vi "HFRR ADV v021 new software.vi"() -> ()   [LabVIEW 2025] (continued)
          tunnel: w1649 -> [w1703 w1716]
          tunnel: w1648 -> [w1702 w1715]
          tunnel: w1647 -> [_ w1714]
          tunnel: w1645 -> [w1688 w1713]
          tunnel: w1644 -> [w1687 w1712]
          tunnel: w1643 -> [w1686 w1711]
          tunnel: [w1688 w1710] -> w1642
          tunnel: [w1687 w1709] -> w1641
          tunnel: [w1686 w1708] -> w1640
          frame False {
          }
          frame True {
            n1436 = Tick Count (ms)() -> (millisecond timer value=w1745:u32)
            n1437 = String To Byte Array(string=w1714) -> (unsigned byte array=w1758:u8[])
            n1438 = Array Size(array=w1758) -> (size(s)=w1757:i32)
            n1439 = formula code="// --- INTERNAL VARIABLE DECLARATIONS ---\nint i = 0;\nint k = 0;\nint start_idx = -1;\nint end_idx = -1;\nint phase = 0;\nint sign0 = 1;\nint sign1 = 1;\nint ch0_val = 0;   \nint ch1_val = 0;   \nfloat ch0_raw = 0.0;\nfloat ch1_raw = 0.0;\nfloat temp0 = 0.0;\nfloat temp1 = 0.0;\nfloat ch0_clean = 0.0;\nfloat ch1_clean = 0.0;\n\n// Temporal intermediate variables for calculation smoothing\nfloat raw_p2p_v = 0.0;\nfloat raw_friction = 0.0;\nfloat raw_cof = 0.0;\n\n// Initialize output variables to current shift register states right away\nout_LVDT_Min_V = in_LVDT_Min_V;\nout_LVDT_Max_V = in_LVDT_Max_V;\nout_LVDT_P2P_V = in_LVDT_P2P_V;\nout_Piezo_P2P = in_Piezo_P2P;\nout_Friction_N = in_Friction_N;\nout_COF = in_COF;\nwindow_ready = 0;\n\n// --- STEP 1: PARSE EVERY STRING IN THE BYTE ARRAY ---\nif (array_size > 2) {\n    for (i = 0; i < array_size - 1; i++) {\n        if (raw_bytes[i] == 42) { // '*' character detected\n            start_idx = i;\n        }\n        \n        // Match standard delimiter sequence \";&\" or end window character\n        if (raw_bytes[i] == 59 && raw_bytes[i+1] == 38 && start_idx != -1) { \n            end_idx = i;\n            ch0_val = 0;\n            ch1_val = 0;\n            sign0 = 1;\n            sign1 = 1;\n            phase = 0; \n\n            for (k = start_idx + 1; k < end_idx; k++) {\n                if (raw_bytes[k] == 45) { // '-' sign\n                    if (phase == 0) sign0 = -1;\n                    else sign1 = -1;\n                }\n                else if (raw_bytes[k] == 43) { // '+' sign\n                    if (phase == 0) sign0 = 1;\n                    else sign1 = 1;\n                }\n                else if (raw_bytes[k] == 59) { // ';' delimiter\n                    phase = 1; \n                }\n                else if (raw_bytes[k] >= 48 && raw_bytes[k] <= 57) { // Numeric ASCII digits\n                    if (phase == 0) {\n                        ch0_val = (ch0_val * 10) + (raw_bytes[k] - 48);\n                    } else {\n                        ch1_val = (ch1_val * 10) + (raw_bytes[k] - 48);\n                    }\n                }\n            }\n\n            // Implicit type conversion\n            ch0_raw = ch0_val * sign0 * 1.0;\n            ch1_raw = ch1_val * sign1 * 1.0;\n\n            // --- STEP 2: 3-SAMPLE MEDIAN FILTER ---\n            m0_2 = m0_1; m0_1 = m0_0; m0_0 = ch0_raw;\n            float s0_0 = m0_0; float s0_1 = m0_1; float s0_2 = m0_2;\n            if (s0_0 > s0_1) { temp0 = s0_0; s0_0 = s0_1; s0_1 = temp0; }\n            if (s0_1 > s0_2) { temp0 = s0_1; s0_1 = s0_2; s0_2 = temp0; }\n            if (s0_0 > s0_1) { temp0 = s0_0; s0_0 = s0_1; s0_1 = temp0; }\n            ch0_clean = s0_1;\n\n            m1_2 = m1_1; m1_1 = m1_0; m1_0 = ch1_raw;\n            float s1_0 = m1_0; float s1_1 = m1_1; float s1_2 = m1_2;\n            if (s1_0 > s1_1) { temp1 = s1_0; s1_0 = s1_1; s1_1 = temp1; }\n            if (s1_1 > s1_2) { temp1 = s1_1; s1_1 = s1_2; s1_2 = temp1; }\n            if (s1_0 > s1_1) { temp1 = s1_0; s1_0 = s1_1; s1_1 = temp1; }\n            ch1_clean = s1_1;\n\n            // --- STEP 3: EXPONENTIAL FILTER (STREAM LEVEL) ---\n            if (ch0_filt == 0.0) ch0_filt = ch0_clean;\n            if (ch1_filt == 0.0) ch1_filt = ch1_clean;\n\n            ch0_filt = ch0_filt + (ch0_clean - ch0_filt) * 0.125;\n            ch1_filt = ch1_filt + (ch1_clean - ch1_filt) * 0.125;\n\n            // --- STEP 4: MIN/MAX WINDOW CONTINUOUS ACCUMULATION ---\n            if (ch0_filt > max_ch0) max_ch0 = ch0_filt;\n            if (ch0_filt < min_ch0) min_ch0 = ch0_filt;\n            if (ch1_filt > max_ch1) max_ch1 = ch1_filt;\n            if (ch1_filt < min_ch1) min_ch1 = ch1_filt;\n\n            start_idx = -1; \n        }\n    }\n}\n\n// --- STEP 5: WINDOW EVALUATION ENGINE ---\nif (((current_time_ms - start_time_ms) >= 50) && (min_ch0 < 9000000.0) && (max_ch0 > -9000000.0)) {\n    window_ready = 1;\n\n    // Linear Bit-to-Voltage Transformations\n    out_LVDT_Min_V = (min_ch0 * VREF) / 8388607.0;\n    out_LVDT_Max_V = (max_ch0 * VREF) / 8388607.0;\n    raw_p2p_v = out_LVDT_Max_V - out_LVDT_Min_V;\n\n    // Piezo scaling calculations\n    out_Piezo_P2P = max_ch1 - min_ch1;\n    raw_friction = out_Piezo_P2P * PIEZO_CAL_FACTOR;\n    raw_cof = raw_friction / NORMAL_FORCE;\n\n    // --- STEP 6: OUTPUT METRIC SMOOTHING (Low-Pass Filter Alpha = 0.20) ---\n    // Seed initial historical metrics if first loop iteration\n    if (hist_LVDT_P2P == 0.0) hist_LVDT_P2P = raw_p2p_v;\n    if (hist_Friction == 0.0) hist_Friction = raw_friction;\n    if (hist_COF == 0.0)      hist_COF = raw_cof;\n\n    // Apply exponential output dampening\n    hist_LVDT_P2P = hist_LVDT_P2P + (raw_p2p_v - hist_LVDT_P2P) * 0.05;\n    hist_Friction = hist_Friction + (raw_friction - hist_Friction) * 0.05;\n    hist_COF      = hist_COF + (raw_cof - hist_COF) * 0.05;\n\n    // Direct smoothed parameters out to UI Indicators\n    out_LVDT_P2P_V = hist_LVDT_P2P;\n    out_Friction_N = hist_Friction;\n    out_COF        = hist_COF;\n\n    // Reset tracking targets to extreme boundaries safely\n    min_ch0 = 9999999.0;\n    max_ch0 = -9999999.0;\n    min_ch1 = 9999999.0;\n    max_ch1 = -9999999.0;\n\n    start_time_ms = current_time_ms;\n}"("raw_bytes"=w1758, "array_size"=w1757, "VREF"="VREF", "PIEZO_CAL_FACTOR"="PIEZO_CAL_FACTOR", "NORMAL_FORCE"="NORMAL_FORCE", "min_ch0"=w1753, "max_ch0"=w1752, "min_ch1"=w1751, "max_ch1"=w1750, "current_time_ms"=w1745, "start_time_ms"=w1744, "ch0_filt"=w1742, "ch1_filt"=w1741, "m0_0"=w1738, "m0_1"=w1737, "m0_2"=w1736, "m1_0"=w1735, "m1_1"=w1734, "m1_2"=w1733, "in_LVDT_Min_V"=w1726, "in_LVDT_Max_V"=w1719, "in_LVDT_P2P_V"=w1718, "in_Piezo_P2P"=w1717, "in_Friction_N"=w1716, "in_COF"=w1715, "hist_LVDT_P2P"=w1713, "hist_Friction"=w1712, "hist_COF"=w1711) -> ("window_ready"=→"Valid_data":dbl, "out_LVDT_Min_V"=w1725:dbl, "out_LVDT_Max_V"=w1724:dbl, "out_LVDT_P2P_V"=w1723:dbl, "out_Piezo_P2P"=w1722:dbl, "out_Friction_N"=w1721:dbl, "out_COF"=w1720:dbl, "min_ch0"=w1749:dbl, "max_ch0"=w1748:dbl, "min_ch1"=w1747:dbl, "max_ch1"=w1746:dbl, "start_time_ms"=w1743:u32, "ch0_filt"=w1740:dbl, "ch1_filt"=w1739:dbl, "m0_0"=w1732:dbl, "m0_1"=w1731:dbl, "m0_2"=w1730:dbl, "m1_0"=w1729:dbl, "m1_1"=w1728:dbl, "m1_2"=w1727:dbl, "hist_LVDT_P2P"=w1710:dbl, "hist_Friction"=w1709:dbl, "hist_COF"=w1708:dbl)
            "LVDT MIN" <- w1725
            "LVDT MAX" <- w1724
            "LVDT Peak" <- w1723
            "pizo raw" <- w1722
            "Friction" <- w1721
            "cof" <- w1720
          }
        }
      }
      frame Error {
      }
    }
    n1440 = local read "Quit"() -> (w1639:bool)
  }
  n1441 = disable-structure shown="Disabled" {
    disable-tunnel: errorcluster {"status"=TRUE, "code"=0, "source"="Init"} ("error IO") -> [w1784 _]
    disable-tunnel: [w1782 _] -> w48
    frame Disabled {
      n1442 = while {
        shift-right: [w1800] -> w1786
        shift-left: _ -> [w1791]
        shift-right: [w1799] -> w1785
        shift-left: w1784 -> [w1793]
        tunnel: [w1788] -> w1782
        tunnel: [w1798] -> _
        i -> [w1798]
        stop <- w1788 stop-if-true
        n1443 = local read "Port 1a"() -> (w1794:bool)
        n1444 = local read "Port 3"() -> (w1795:bool)
        n1445 = local read "Com Port 1"() -> (w1792:refnum<visa-resource-name>)
        n1446 = Or(x=w1795, y=w1794) -> (x .or. y?=w1797:bool)
        n1447 = Unbundle(w1793) -> ("status"=→"Port 3":bool)  [unwired: 2 out]
        n1448 = Not Equal?(x=w1792, y=w1791) -> (x != y?=w1789:bool)
        n1449 = case shown="True" w1797 {
          frame False {
            w1803 = TRUE ("Visible")
            n1450 = property on="Port 1a" class="Bool (strict)"("Visible"=w1803) -> ()  [unwired: 2 in, 2 out]
            n1451 = property on="Port 3" class="Bool (strict)"("Visible"=w1803) -> ()  [unwired: 2 in, 2 out]
          }
          frame True {
            w1804 = TRUE ("Visible")
            n1452 = property on="Port 1a" class="Bool (strict)"("Visible"=w1804) -> ()  [unwired: 2 in, 2 out]
            n1453 = property on="Port 3" class="Bool (strict)"("Visible"=w1804) -> ()  [unwired: 2 in, 2 out]
          }
        }
        n1454 = Wait (ms)(milliseconds to wait=u32 40) -> ()  [unwired: 1 out]
        n1455 = case shown="True" w1789 {
          tunnel: [w1801 errorcluster {"status"=TRUE, "code"=0, "source"="Init"} ("error out")] -> w1790
          tunnel: w1793 -> [w1801 _]
          frame False {
          }
          frame True {
          }
        }
        "error out 11" <- w1790
        n1456 = case shown="No Error" w1790 {
          selector: w1790 -> [w1811 w1829]
          tunnel: [w1814 w1833] -> w1800
          tunnel: [w1813 w1827] -> w1799
          tunnel: w1791 -> [w1812 w1831]
          frame No Error {
            n1457 = property class="Instr"(reference=w1812, error in=w1811) -> (reference out=w1809:refnum<visa-resource-name>, error out=w1810:errorcluster, "Serial Settings:Number of Bytes at Serial Port"=w1806:u32)
            n1458 = Greater?(x=w1806, y=u32 5) -> (0:w1805:bool)
            n1459 = Not(x=w1805) -> (.not. x?=→"Port 1a":bool)
            n1460 = while {
              tunnel: [w1822] -> w1813
              tunnel: [w1821] -> w1814
              tunnel: w1810 -> [w1820]
              tunnel: w1809 -> [w1819]
              stop <- TRUE stop-if-true
              n1461 = property class="Instr" props=["Serial Settings:Number of Bytes at Serial Port"](reference=w1819, error in=w1820) -> (reference out=w1824:refnum<visa-resource-name>, error out=w1823:errorcluster)  [unwired: 1 out]
              n1462 = VISA Read(VISA resource name=w1824, byte count=u32 50, error in (no error)=w1823) -> (VISA resource name out=w1821:refnum<visa-resource-name>, read buffer=→"UNI READ":string, error out=w1822:errorcluster)  [unwired: 1 out]
              n1463 = Wait (ms)(milliseconds to wait=u32 5) -> ()  [unwired: 1 out]
            }
          }
          frame Error {
            w1839 = u16 0 items=["None", "XON/XOFF", "RTS/CTS", "XON/XOFF & RTS/CTS", "DTR/DSR", "XON/XOFF & DTR/DSR"] ("flow control (0:none)  2")
            w1837 = u16 10 items=["1.0"=10, "1.5"=15, "2.0"=20] ("stop bits 2")
            w1835 = u16 0 items=["None", "Odd", "Even", "Mark", "Space"] ("parity 2")
            w1836 = u32 10000  # timeout (10sec)
            n1464 = VISA Close(VISA resource name=w1831, error in (no error)=w1829) -> (error out=w1832:errorcluster)
            n1465 = local write "Port 1a"(FALSE ("Port 1a")) -> ()
            n1466 = local read "Com Port 1"() -> (w1826:refnum<visa-resource-name>)
            n1467 = call <vilib>:"Clear Errors.vi"("error in (no error)"=w1832) -> ("error out"=w1830:errorcluster)  [unwired: 5 in, 1 out]
            n1468 = call-poly "VISA Configure Serial Port"("VISA resource name"=w1826, "timeout (10sec)"=w1836, "baud rate (9600)"=u32 250000 ("baud rate  2"), "data bits (8)"=u16 8 ("data bits  2"), "parity (0:none)"=w1835, "error in (no error)"=w1830, "stop bits (10: 1 bit)"=w1837, "flow control (0:none)"=w1839) -> ("VISA resource name out"=w1840:refnum<visa-resource-name>, "error out"=w1841:errorcluster)  [unwired: 6 in]
            n1469 = flat-sequence {
              tunnel: w1840 -> [w1843]
              tunnel: w1841 -> [w1842]
              tunnel: [w1843] -> w1833
              tunnel: [w1842] -> w1827
              frame #0 {
                n1470 = Wait (ms)(milliseconds to wait=u32 50) -> ()  [unwired: 1 out]
              }
            }
            "Residual Uno" <- ""
            "Port 1 Error" <- w1827
          }
        }
        n1471 = local read "Quit"() -> (w1788:bool)
        "Error Uno" <- w1793
      }
      n1472 = VISA Close(VISA resource name=w1786, error in (no error)=w1785) -> (error out=w1783:errorcluster)
      n1473 = call <vilib>:"Clear Errors.vi"("error in (no error)"=w1783) -> ()  [unwired: 5 in, 2 out]
    }
    frame Enabled {
    }
  }
  n1474 = while {
    stop <- w1854 stop-if-true
    # "V0OLTAGE TO STROKE (peice vise calibration)"
    n1475 = local read "LVDT MIN"() -> (w1845:dbl)
    n1476 = Wait (ms)(milliseconds to wait=u32 10) -> ()  [unwired: 1 out]
    n1477 = local read "LVDT Peak"() -> (w1846:dbl)
    n1478 = formula code="// Dynamic Parameterized Linear Interpolation Node\n// Inputs: vpp_val, voltages (Array), distances (Array)\n// Outputs: stroke\n\nint i = 0;\nint segments = 11; // 12 points make 11 interpolation segments\n\n// 1. Lower Boundary Clamp\nif (vpp_val <= voltages[0]) {\n    stroke = distances[0];\n}\n// 2. Upper Boundary Clamp\nelse if (vpp_val >= voltages[segments]) {\n    stroke = distances[segments];\n}\n// 3. Dynamic Segment Search Loop\nelse {\n    stroke = distances[0]; // Fallback baseline\n    for (i = 0; i < segments; i++) {\n        if (vpp_val >= voltages[i] && vpp_val <= voltages[i+1]) {\n            // Standard linear interpolation formula using array lookups\n            stroke = distances[i] + (vpp_val - voltages[i]) * (distances[i+1] - distances[i]) / (voltages[i+1] - voltages[i]);\n            break; // Segment found, safely exit the loop\n        }\n    }\n}"("vpp_val"=w1846, "voltages"="calibration values", "distances"="STROKE") -> ("stroke"=→"LVDT STROKE":dbl)
    n1479 = local read "Calibration Tare Value"() -> (w1850:dbl)
    n1480 = local read "Calibration Tare"() -> (w1848:bool)
    n1481 = Subtract(x=w1845, y=w1850) -> (x-y=→"LVDT STROKE  Calibration":dbl)
    n1482 = case shown="True" w1848 {
      selector: w1848 -> [_ w1856]
      tunnel: w1845 -> [_ w1857]
      frame False {
      }
      frame True {
        n1483 = Not(x=w1856) -> (.not. x?=w1855:bool)
        n1484 = local write "Calibration Tare"(w1855) -> ()
        "Calibration Tare Value" <- w1857
      }
    }
    n1485 = local read "Quit"() -> (w1854:bool)
  }
  n1486 = while {
    stop <- w1877 stop-if-true
    n1487 = call <vilib>:"High Resolution Polling Wait.vi"("seconds to wait"=0.02) -> ()  [unwired: 10 in, 1 out]
    n1488 = local read "Due read"() -> (w1875:string)
    n1489 = Spreadsheet String To Array(delimiter (Tab)=";", format string="", spreadsheet string=w1875, array type (2D Dbl)=string[] []) -> (array=w1872:string[])
    n1490 = Fract/Exp String To Number(string=w1872) -> (number=w1871:dbl[])  [unwired: 3 in, 1 out]
    n1491 = Index Array(array=w1871) -> (element #1=→"Sample Temperature":dbl, element #2=→"Target Sample Temperature":dbl, element #3=→"Current Duty Cycle":dbl, element #4=→"Ambient Temperature":dbl, element #5=→"Dac Status":dbl, element #6=→"Vpp":dbl, element #7=→"Active Error Code":dbl, element #8=→"Kp":dbl, element #9=→"Ki":dbl, element #10=→"Kd":dbl, element #11=→"SampleRaw":dbl, element #12=→"AmbRaw":dbl)  [unwired: 12 in]
    n1492 = local read "Quit"() -> (w1877:bool)
  }
  n1493 = while {
    shift-right: [w1891] -> w43
    shift-left: _ -> [w1882]
    shift-right: [w1890] -> w42
    shift-left: errorcluster {"status"=FALSE, "code"=0, "source"="Init"} ("error out") -> [w1884]
    tunnel: [w1879] -> w47
    tunnel: [w1889] -> _
    i -> [w1889]
    stop <- w1879 stop-if-true
    n1494 = local read "Com Port 2"() -> (w1883:refnum<visa-resource-name>)
    n1495 = local read "Port 2a"() -> (w1885:bool)
    n1496 = Unbundle(w1884) -> ("status"=→"Port 4":bool)  [unwired: 2 out]
    n1497 = call <vilib>:"High Resolution Polling Wait.vi"("seconds to wait"=0.02) -> ()  [unwired: 10 in, 1 out]
    n1498 = local read "Port 4"() -> (w1886:bool)
    n1499 = Not Equal?(x=w1883, y=w1882) -> (x != y?=w1881:bool)
    n1500 = Or(x=w1886, y=w1885) -> (x .or. y?=w1888:bool)
    n1501 = case shown="False" w1888 {
      frame False {
        w1894 = TRUE ("Visible")
        n1502 = property on="Port 2a" class="Bool (strict)"("Visible"=w1894) -> ()  [unwired: 2 in, 2 out]
        n1503 = property on="Port 4" class="Bool (strict)"("Visible"=w1894) -> ()  [unwired: 2 in, 2 out]
      }
      frame True {
        w1895 = TRUE ("Visible")
        n1504 = property on="Port 2a" class="Bool (strict)"("Visible"=w1895) -> ()  [unwired: 2 in, 2 out]
        n1505 = property on="Port 4" class="Bool (strict)"("Visible"=w1895) -> ()  [unwired: 2 in, 2 out]
      }
    }
    n1506 = case shown="True" w1881 {
      tunnel: [w1892 errorcluster {"status"=TRUE, "code"=0, "source"="Init"} ("error out")] -> w1880
      tunnel: w1884 -> [w1892 _]
      frame False {
      }
      frame True {
      }
    }
    n1507 = case shown="No Error" w1880 {
      selector: w1880 -> [w1908 w1939]
      tunnel: [w1901 w1944] -> w1891
      tunnel: [w1909 w1937] -> w1890
      tunnel: w1882 -> [w1910 w1942]
      frame No Error {
        n1508 = property class="Instr" props=["Serial Settings:Number of Bytes at Serial Port"](reference=w1910, error in=w1908) -> (reference out=w1902:refnum<visa-resource-name>, error out=w1907:errorcluster)  [unwired: 1 out]
        n1509 = while {
          tunnel: [w1918] -> w1903
          tunnel: [w1917] -> w1904
          tunnel: w1907 -> [w1916]
          tunnel: w1902 -> [w1915]
          tunnel: [w1914] -> _
          i -> [w1914]
          stop <- TRUE stop-if-true
          n1510 = property class="Instr" props=["Serial Settings:Number of Bytes at Serial Port"](reference=w1915, error in=w1916) -> (reference out=w1920:refnum<visa-resource-name>, error out=w1919:errorcluster)  [unwired: 1 out]
          n1511 = VISA Read(VISA resource name=w1920, byte count=u32 1000, error in (no error)=w1919) -> (VISA resource name out=w1917:refnum<visa-resource-name>, read buffer=→"Due read":string, error out=w1918:errorcluster)  [unwired: 1 out]
        }
        n1512 = local read "Command"() -> (w1900:string)
        n1513 = call <vilib>:"Trim Whitespace.vi"("string"=w1900) -> ("trimmed string"=w1899:string)  [unwired: 1 in]
        n1514 = Not Equal?(x=w1899, y="") -> (x != y?=w1905:bool)
        n1515 = VISA Flush I/O Buffer(VISA resource name=w1904) -> (VISA resource name out=w1897:refnum<visa-resource-name>, error out=→"error out 10":errorcluster)  [unwired: 2 in]
        n1516 = case shown="True" w1905 {
          tunnel: w1897 -> [w1922 w1927]
          tunnel: [w1922 w1931] -> w1901
          tunnel: w1903 -> [w1921 w1926]
          tunnel: [w1921 w1929] -> w1909
          tunnel: w1899 -> [_ w1925]
          tunnel: [_ w1928] -> _
          frame False {
            # "DATA  WRITE LOOP"
          }
          frame True {
            n1517 = Concatenate Strings(w1925, "\r\n") -> (w1924:string)
            n1518 = VISA Write(VISA resource name=w1927, write buffer=w1924, error in (no error)=w1926) -> (VISA resource name out=w1931:refnum<visa-resource-name>, return count=w1928:u32, error out=w1930:errorcluster)
            n1519 = flat-sequence {
              tunnel: w1930 -> [w1933]
              tunnel: [w1933] -> w1929
              frame #0 {
                n1520 = local write "Command"("" ("Command")) -> ()
                n1521 = Wait (ms)(milliseconds to wait=u32 5) -> ()  [unwired: 1 out]
              }
            }
          }
        }
        "Port 2a" <- TRUE ("Port 2a")
      }
      frame Error {
        w1950 = u16 0 items=["None", "XON/XOFF", "RTS/CTS", "XON/XOFF & RTS/CTS", "DTR/DSR", "XON/XOFF & DTR/DSR"] ("flow control (0:none)  2")
        w1948 = u16 10 items=["1.0"=10, "1.5"=15, "2.0"=20] ("stop bits 2")
        w1946 = u16 0 items=["None", "Odd", "Even", "Mark", "Space"] ("parity 2")
        w1947 = u32 10000  # timeout (10sec)
        n1522 = VISA Clear(VISA resource name=w1942, error in (no error)=w1939) -> (VISA resource name out=w1941:refnum<visa-resource-name>, error out=w1940:errorcluster)
        n1523 = VISA Close(VISA resource name=w1941, error in (no error)=w1940) -> (error out=w1943:errorcluster)
        n1524 = call <vilib>:"Clear Errors.vi"("error in (no error)"=w1943) -> ()  [unwired: 5 in, 2 out]
        n1525 = local write "Port 2a"(FALSE ("Port 2a")) -> ()
        n1526 = local read "Com Port 2"() -> (w1936:refnum<visa-resource-name>)
        "visa due" <- w1936
        n1527 = call-poly "VISA Configure Serial Port"("VISA resource name"=w1936, "timeout (10sec)"=w1947, "baud rate (9600)"=u32 250000 ("baud rate  2"), "data bits (8)"=u16 8 ("data bits  2"), "parity (0:none)"=w1946, "stop bits (10: 1 bit)"=w1948, "flow control (0:none)"=w1950) -> ("VISA resource name out"=w1951:refnum<visa-resource-name>, "error out"=w1952:errorcluster)  [unwired: 7 in]
        n1528 = flat-sequence {
          tunnel: w1951 -> [w1954]
          tunnel: w1952 -> [w1953]
          tunnel: [w1954] -> w1944
          tunnel: [w1953] -> w1937
          frame #0 {
            n1529 = Wait (ms)(milliseconds to wait=u32 50) -> ()  [unwired: 1 out]
          }
        }
        "Residual Due" <- ""
        "Port 2 Error" <- w1937
      }
    }
    n1530 = local read "Quit"() -> (w1879:bool)
    "Error Due" <- w1884
  }
  n1531 = local write "FRICVALZ"(0.0 ("FRICVALZ")) -> ()
  n1532 = property on="RUN" class="Bool (strict)"("Visible"=TRUE) -> ()  [unwired: 2 in, 2 out]
  n1533 = while {
    tunnel: [w1971] -> _
    tunnel: [w1956] -> w57
    i -> [w1971]
    stop <- w1956 stop-if-true
    n1534 = local read "conststatus"() -> (w1960:dbl)
    n1535 = local read "Main Tab"() -> (w1958:T2)
    n1536 = local read "EDIT"() -> (w1977:bool)
    n1537 = local read "Rate"() -> (w1976:dbl)
    n1538 = case shown="True" w1977 {
      tunnel: [FALSE TRUE] -> w1963
      frame False {
      }
      frame True {
      }
    }
    n1539 = property on="Time slide" class="Slide (strict)"("Scale.Range:Maximum"=2500.0) -> ()  [unwired: 2 in, 2 out]
    n1540 = Equal?(x=w1958, y=T27."About" ("Main Tab")) -> (x = y?=w1969:bool)
    n1541 = Equal?(x=w1960, y=0.0) -> (x = y?=w1961:bool)
    n1542 = Divide(x=1.0, y=w1976) -> (x/y=w1972:dbl)
    "Time 2" <- w1972
    n1543 = case shown="True" w1961 {
      frame False {
      }
      frame True {
        # "C:\\WinDucom\\calibrate WO 2391.dcf"
        n1544 = local write "Lan flag"(22) -> ()
        n1545 = local write "conststatus"(10.0 ("rpm value : 2")) -> ()
        n1546 = String To Path(string="C:\\LAB-IQ\\calibrate WO 2465.dcf") -> (path=w1983:path)
        n1547 = Open/Create/Replace File "Open File"(file path (use dialog)=w1983) -> (refnum out=w1981:refnum<file>)  [unwired: 5 in, 2 out]
        n1548 = for {
          N: 23 -> [_]
          tunnel: w1981 -> [w1992]
          i -> [w1986]
          (unwired) TRUE ("line mode (F)")
          n1549 = Read from Text File "Read File"(file (use dialog)=w1992) -> (text=w1991:string)  [unwired: 3 in, 3 out]
          n1550 = Match Pattern(string=w1991, regular expression="]") -> (after substring=w1989:string)  [unwired: 1 in, 3 out]
          n1551 = String Subset(string=w1991, offset (0)=5, length (rest)=10 ("length (rest)")) -> (substring=w1984:string)
          n1552 = Fract/Exp String To Number(string=w1984) -> (number=w1985:dbl)  [unwired: 3 in, 1 out]
          n1553 = Match Pattern(string=w1989, regular expression="-") -> (before substring=w1987:string)  [unwired: 1 in, 3 out]
          n1554 = case shown="4" w1986 {
            tunnel: w1985 -> [w1995 w1996 w1997 w1998 _ _ _ w2003 w2004 _ w2005 w2006 w2007 w2008 w2009 w2010 _ w2011 w2012 _ _ _ _ _]
            tunnel: w1987 -> [_ _ _ _ w1999 w2000 w2001 _ _ _ _ _ _ _ _ _ _ _ _ w2013 w2014 w2015 w2016 _]
            frame 0 {
              n1555 = local write "FRIC. FORCE :"(w1995) -> ()
            }
            frame 1 {
              n1556 = local write "TEMPERATURE :"(w1996) -> ()
            }
            frame 2 {
              n1557 = local write "HUMIDITY:"(w1997) -> ()
            }
            frame 3 {
              n1558 = local write "AIR TEMPERATURE :"(w1998) -> ()
            }
            frame 4 {
              n1559 = local write "Com Port 1"(w1999) -> ()
            }
            frame 5 {
              n1560 = local write "Com Port 2"(w2000) -> ()
              n1561 = local write "visa due"(w2000) -> ()
            }
            frame 6 {
              n1562 = String To Path(string=w2001) -> (path=w2002:path)
              n1563 = local write "File Path"(w2002) -> ()
              "String" <- w2001
            }
            frame 7 {
              n1564 = local write "DISPLACEMENT :"(w2003) -> ()
            }
            frame 8 {
              n1565 = local write "STROKE GAIN :"(w2004) -> ()
            }
            frame 9 {
            }
            frame 10 {
              n1566 = local write "Language Selection"(w2005) -> ()
            }
            frame 11 {
              n1567 = local write "CH-POWER +"(w2006) -> ()
            }
            frame 12 {
              n1568 = local write "CH-POWER -"(w2007) -> ()
            }
            frame 13 {
              n1569 = local write "CH-HEATER"(w2008) -> ()
            }
            frame 14 {
              n1570 = local write "CH-HUMIDITY WET"(w2009) -> ()
            }
            frame 15 {
              n1571 = local write "CH-HUMIDITY DRY"(w2010) -> ()
            }
            frame 16 {
            }
            frame 17 {
              n1572 = local write "AIR TEMP INTERCEPT:"(w2011) -> ()
            }
            frame 18 {
              n1573 = local write "TEMP INTERCEPT:"(w2012) -> ()
            }
            frame 21 {
              n1574 = local write "S.NO"(w2013) -> ()
            }
            frame 22 {
              n1575 = local write "Com Port 3"(w2014) -> ()
            }
            frame 20 {
              n1576 = local write "Camera Port :"(w2015) -> ()
            }
            frame 19 {
              n1577 = local write "C3 :"(w2016) -> ()
            }
            frame 23, Default {
            }
          }
        }
      }
    }
    n1578 = Select(t=u32 2500 ("milliseconds to wait"), s=w1969, f=u32 500 ("milliseconds to wait")) -> (s? t:f=w1967:u32)
    n1579 = Multiply(x=w1972, y=w1967) -> (x*y=w1974:dbl)
    n1580 = property on="Time slide" class="Slide (strict)"("Visible"=w1963) -> ()  [unwired: 2 in, 2 out]
    n1581 = call "Elapsed Time2"("Time Target (s)"=w1974, "Auto Reset"=TRUE) -> ("Time has Elapsed"=w1964:bool)  [unwired: 10 in, 7 out]
    n1582 = case shown="True" w1964 {
      frame False {
      }
      frame True {
        n1583 = stacked-sequence {
          frame #0 {
            # "DATA PROCESSING"
            # "115 mV/N"
            n1584 = local read "Sample Temperature"() -> (w2019:dbl)
            n1585 = local read "RH Numeric:"() -> (w2026:dbl)
            n1586 = local read "HUMIDITY:"() -> (w2027:dbl)
            n1587 = local read "FRICVALZ"() -> (w2038:dbl)
            n1588 = local read "Friction"() -> (w2022:dbl)
            n1589 = Multiply(x=w2026, y=w2027) -> (x*y=→"Humidity ( %RH )" →"Hum" →"Hum 2":dbl)
            n1590 = call <vilib>:"Mean PtByPt.vi"("x"=w2019, "sample length"=100) -> ("mean"=w2018:dbl)  [unwired: 2 in, 1 out]
            "TEMP 2" <- w2018
            "TEMP 3" <- w2018
            n1591 = Subtract(x=w2022, y=w2038) -> (x-y=w2033:dbl)
            "FF 2" <- w2033
            "FF 4" <- w2033
            n1592 = local read "Ambient Temperature"() -> (→"AIR TEMP":dbl)
            n1593 = local read "TEMP"() -> (w2037:dbl)
            n1594 = local write "FF 3"(w2033) -> ()
            n1595 = Compound Arithmetic op=OR("FRICVALZ 4", "FRICVALZ 3", "FRICVALZ 2") -> (w2029:bool)
            n1596 = case shown="True" w2029 {
              tunnel: w2022 -> [_ w2044]
              frame False {
              }
              frame True {
                w2043 = FALSE ("FRICVALZ")
                n1597 = local write "FRICVALZ 3"(w2043) -> ()
                n1598 = local write "FRICVALZ 2"(w2043) -> ()
                n1599 = local write "FRICVALZ 4"(w2043) -> ()
                "FRICVALZ" <- w2044
              }
            }
            n1600 = Not A Number/Path/Refnum?(number/path/refnum=w2037) -> (NaN/Path/Refnum?=w2036:bool)
            n1601 = Not A Number/Path/Refnum?(number/path/refnum=w2033) -> (NaN/Path/Refnum?=w2035:bool)
            n1602 = Divide(x=w2033, y=1.96) -> (x/y=w2030:dbl)
            n1603 = Compound Arithmetic op=OR(w2036, w2035) -> (w2034:bool)
            n1604 = Not A Number/Path/Refnum?(number/path/refnum=w2030) -> (NaN/Path/Refnum?=w2031:bool)
            n1605 = case shown="True" w2034 {
              frame False {
              }
              frame True {
                n1606 = local write "TEMP"(0.0 ("TEMP")) -> ()
                n1607 = local write "FF 2"(0.0 ("FF 2")) -> ()
                n1608 = local write "reinit"(TRUE ("reinit")) -> ()
              }
            }
            n1609 = local write "TEMP"(w2018) -> ()
            n1610 = Select(t=0.0, s=w2031, f=w2030) -> (s? t:f=w2021:dbl)
            "COF 2" <- w2021
            n1611 = local write "COF 3"(w2021) -> ()
          }
        }
      }
    }
    n1612 = Wait (ms)(milliseconds to wait=u32 50) -> ()  [unwired: 1 out]
    n1613 = local read "Quit"() -> (w1956:bool)
    "Rate" <- 2500.0 ("No of Samples")
  }
  n1614 = while {
    tunnel: w60 -> [_]
    tunnel: [w2071] -> _
    tunnel: [w2047] -> w59
    i -> [w2071]
    stop <- w2047 stop-if-true
    # "C:\\LAB-IQ-NXT\\Scar View.exe"
    n1615 = local read "OK Button 16"() -> (w2060:bool)
    n1616 = local read "Main Tab"() -> (w2053:T2)
    n1617 = local read "service 3"() -> (w2054:bool)
    n1618 = local read "OPEN 6"() -> (w2056:bool)
    n1619 = local read "EDIT 2"() -> (w2058:bool)
    n1620 = flat-sequence {
      frame #0 {
        n1621 = local read "SAVE 2"() -> (w2673:bool)
        n1622 = stacked-sequence {
          frame #0 {
            n1623 = local read "EDIT"() -> (w2727:bool)
            n1624 = case shown="True" w2727 {
              tunnel: [u8 2 ("Disabled") u8 0 ("Disabled")] -> _
              frame False {
                w2729 = FALSE
                n1625 = local write "Password"("") -> ()
                n1626 = property on="SrvM CP" class="Bool (strict)"("Visible"=w2729) -> ()  [unwired: 2 in, 2 out]
                n1627 = property on="message" class="Str"("Visible"=w2729) -> ()  [unwired: 2 in, 2 out]
                n1628 = local write "x = y?"(w2729) -> ()
                n1629 = property on="Password" class="Str"("Visible"=w2729) -> ()  [unwired: 2 in, 2 out]
                n1630 = property on="ENTER THE NEW PASSWORD" class="Str"("Visible"=w2729) -> ()  [unwired: 2 in, 2 out]
                n1631 = property on="ENTER CURRENT PASSWORD" class="Str"("Visible"=w2729) -> ()  [unwired: 2 in, 2 out]
                n1632 = local write "SrvM CP"(w2729) -> ()
              }
              frame True {
                w2732 = TRUE
                n1633 = property on="SrvM CP" class="Bool (strict)"("Visible"=w2732) -> ()  [unwired: 2 in, 2 out]
                n1634 = property on="Password" class="Str"("Visible"=w2732) -> ()  [unwired: 2 in, 2 out]
              }
            }
            "dipl pwd" <- "@143$\n" ("dipl pwd")
          }
          frame #1 {
            # "Gain password"
            n1635 = String To Byte Array(string="ENTER CURRENT PASSWORD") -> (unsigned byte array=w2737:u8[])
            n1636 = Search 1D Array(1D array=w2737, element=u8 10) -> (index of element=w2740:i32)  [unwired: 1 in]
            n1637 = Index Array(array=w2737, index=w2740) -> (element=w2736:u8)
            n1638 = Equal?(x=w2736, y=10) -> (x = y?=w2734:bool)
            n1639 = case shown="True" w2734 {
              frame False {
                n1640 = property on="ENTER THE NEW PASSWORD" class="Str"("Visible"=FALSE) -> ()  [unwired: 2 in, 2 out]
              }
              frame True {
                # "password"
                # "change password logic"
                n1641 = local read "ENTER CURRENT PASSWORD"() -> (w2753:string)
                n1642 = local read "dipl pwd"() -> (w2747:string)
                n1643 = String To Byte Array(string=w2753) -> (unsigned byte array=w2755:u8[])
                n1644 = String To Byte Array(string=w2747) -> (unsigned byte array=w2748:u8[])
                n1645 = Array Size(array=w2755) -> (size(s)=w2752:i32)
                n1646 = Array Size(array=w2748) -> (size(s)=w2750:i32)
                n1647 = for {
                  N: w2752 -> [_]
                  tunnel: w2755 -> [w2779]
                  tunnel: [w2777] -> w2756 mode=indexing
                  tunnel: w2752 -> [w2771]
                  i -> [w2772]
                  n1648 = Decrement(x=w2771) -> (x-1=w2769:i32)
                  n1649 = Equal?(x=w2772, y=w2769) -> (x = y?=w2770:bool)
                  n1650 = Index Array(array=w2779, index=w2772) -> (element=w2773:u8)
                  n1651 = Number To Decimal String(number=w2773) -> (decimal integer string=w2778:string)  [unwired: 1 in]
                  n1652 = Select(t="", s=w2770, f="\r") -> (s? t:f=w2775:string)
                  n1653 = Concatenate Strings(w2778, w2775) -> (w2777:string)
                }
                n1654 = for {
                  N: w2750 -> [_]
                  tunnel: w2748 -> [w2767]
                  tunnel: [w2765] -> w2749 mode=indexing
                  tunnel: w2750 -> [w2762]
                  i -> [w2763]
                  n1655 = Decrement(x=w2762) -> (x-1=w2761:i32)
                  n1656 = Equal?(x=w2763, y=w2761) -> (x = y?=w2760:bool)
                  n1657 = Index Array(array=w2767, index=w2763) -> (element=w2766:u8)
                  n1658 = Number To Decimal String(number=w2766) -> (decimal integer string=w2764:string)  [unwired: 1 in]
                  n1659 = Select(t="", s=w2760, f="\r") -> (s? t:f=w2757:string)
                  n1660 = Concatenate Strings(w2764, w2757) -> (w2765:string)
                }
                n1661 = local read "string"() -> (w2754:string)
                n1662 = Concatenate Strings(w2749) -> (w2743:string)
                n1663 = Concatenate Strings(w2754) -> (w2751:string)
                n1664 = Concatenate Strings(w2756) -> (w2744:string)
                n1665 = Equal?(x=w2744, y=w2751) -> (x = y?=w2746:bool)
                n1666 = Equal?(x=w2744, y=w2743) -> (x = y?=w2742:bool)
                n1667 = Or(x=w2746, y=w2742) -> (x .or. y?=w2745:bool)
                n1668 = case shown="True" w2745 {
                  frame False {
                  }
                  frame True {
                    n1669 = property on="ENTER THE NEW PASSWORD" class="Str"("Visible"=TRUE) -> ()  [unwired: 2 in, 2 out]
                  }
                }
              }
            }
          }
          frame #2 {
            n1670 = String To Byte Array(string="ENTER THE NEW PASSWORD") -> (unsigned byte array=w2782:u8[])
            n1671 = Search 1D Array(1D array=w2782, element=u8 10) -> (index of element=w2786:i32)  [unwired: 1 in]
            n1672 = Index Array(array=w2782, index=w2786) -> (element=w2784:u8)
            n1673 = Equal?(x=w2784, y=10) -> (x = y?=w2781:bool)
            n1674 = case shown="False" w2781 {
              frame False {
              }
              frame True {
                n1675 = local write "EDIT"(FALSE) -> ()
                n1676 = local write "SrvM CP"(FALSE) -> ()
                n1677 = local read "ENTER THE NEW PASSWORD"() -> (w2789:string)
                n1678 = String To Byte Array(string=w2789) -> (unsigned byte array=w2794:u8[])
                n1679 = Array Size(array=w2794) -> (size(s)=w2791:i32)
                n1680 = for {
                  N: w2791 -> [_]
                  tunnel: w2794 -> [w2807]
                  tunnel: [w2804] -> w2796 mode=indexing
                  tunnel: w2791 -> [w2799]
                  i -> [w2797]
                  n1681 = Decrement(x=w2799) -> (x-1=w2800:i32)
                  n1682 = Equal?(x=w2797, y=w2800) -> (x = y?=w2801:bool)
                  n1683 = Index Array(array=w2807, index=w2797) -> (element=w2806:u8)
                  n1684 = Number To Decimal String(number=w2806) -> (decimal integer string=w2805:string)  [unwired: 1 in]
                  n1685 = Select(t="", s=w2801, f="\r") -> (s? t:f=w2798:string)
                  n1686 = Concatenate Strings(w2805, w2798) -> (w2804:string)
                }
                n1687 = local read "file path"() -> (w2788:path)
                n1688 = Concatenate Strings(w2796) -> (w2790:string)
                n1689 = Delete(path (use dialog)=w2788) -> (deleted path=w2792:path)  [unwired: 4 in, 2 out]
                n1690 = call <vilib>:"Write Characters To File.vi"("append to file? (new file:F)"=FALSE, "character string"=w2790, "file path (dialog if empty)"=w2792) -> ()  [unwired: 2 in, 1 out]
              }
            }
          }
          frame #3 {
            n1691 = case shown="True" "SrvM CP" {
              frame False {
                w2810 = ""
                n1692 = local write "ENTER CURRENT PASSWORD"(w2810) -> ()
                n1693 = local write "ENTER THE NEW PASSWORD"(w2810) -> ()
                n1694 = property on="ENTER CURRENT PASSWORD" class="Str"("Visible"=FALSE) -> ()  [unwired: 2 in, 2 out]
              }
              frame True {
                n1695 = property on="ENTER THE NEW PASSWORD" class="Str"() -> ("Visible"=w2811:bool)  [unwired: 2 in, 2 out]
                n1696 = Not(x=w2811) -> (.not. x?=w2812:bool)
                n1697 = property on="ENTER CURRENT PASSWORD" class="Str"("Visible"=w2812) -> ()  [unwired: 2 in, 2 out]
              }
            }
          }
          frame #4 {
            n1698 = String To Byte Array(string="Password") -> (unsigned byte array=w2819:u8[])
            n1699 = Search 1D Array(1D array=w2819, element=u8 10) -> (index of element=w2817:i32)  [unwired: 1 in]
            n1700 = Index Array(array=w2819, index=w2817) -> (element=w2818:u8)
            n1701 = Equal?(x=w2818, y=10) -> (x = y?=w2814:bool)
            n1702 = case shown="True" w2814 {
              frame False {
              }
              frame True {
                # "password"
                # "password"
                n1703 = local read "Password"() -> (w2832:string)
                n1704 = String To Byte Array(string=w2832) -> (unsigned byte array=w2835:u8[])
                n1705 = String To Byte Array(string="@143$\n") -> (unsigned byte array=w2821:u8[])
                n1706 = Array Size(array=w2835) -> (size(s)=w2830:i32)
                n1707 = Array Size(array=w2821) -> (size(s)=w2826:i32)
                n1708 = for {
                  N: w2830 -> [_]
                  tunnel: w2835 -> [w2869]
                  tunnel: [w2867] -> w2836 mode=indexing
                  tunnel: w2830 -> [w2864]
                  i -> [w2865]
                  n1709 = Decrement(x=w2864) -> (x-1=w2863:i32)
                  n1710 = Index Array(array=w2869, index=w2865) -> (element=w2868:u8)
                  n1711 = Equal?(x=w2865, y=w2863) -> (x = y?=w2862:bool)
                  n1712 = Number To Decimal String(number=w2868) -> (decimal integer string=w2866:string)  [unwired: 1 in]
                  n1713 = Select(t="", s=w2862, f="\r") -> (s? t:f=w2859:string)
                  n1714 = Concatenate Strings(w2866, w2859) -> (w2867:string)
                }
                n1715 = for {
                  N: w2826 -> [_]
                  tunnel: w2821 -> [w2880]
                  tunnel: [w2878] -> w2824 mode=indexing
                  tunnel: w2826 -> [w2875]
                  i -> [w2876]
                  n1716 = Decrement(x=w2875) -> (x-1=w2874:i32)
                  n1717 = Index Array(array=w2880, index=w2876) -> (element=w2879:u8)
                  n1718 = Equal?(x=w2876, y=w2874) -> (x = y?=w2873:bool)
                  n1719 = Number To Decimal String(number=w2879) -> (decimal integer string=w2877:string)  [unwired: 1 in]
                  n1720 = Select(t="", s=w2873, f="\r") -> (s? t:f=w2870:string)
                  n1721 = Concatenate Strings(w2877, w2870) -> (w2878:string)
                }
                n1722 = local read "file path"() -> (w2820:path)
                n1723 = call <vilib>:"Read Characters From File.vi"("file path (dialog if empty)"=w2820) -> ("character string"=w2834:string)  [unwired: 5 in, 3 out]
                "string" <- w2834
                n1724 = flat-sequence {
                  tunnel: [w2837] -> w2831
                  frame #0 {
                    w2837 = ""
                    n1725 = local write "Password"(w2837) -> ()
                  }
                }
                n1726 = Concatenate Strings(w2824) -> (w2825:string)
                n1727 = Concatenate Strings(w2834) -> (w2833:string)
                n1728 = Concatenate Strings(w2836) -> (w2828:string)
                n1729 = Equal?(x=w2828, y=w2833) -> (x = y?=w2823:bool)
                n1730 = Equal?(x=w2828, y=w2825) -> (x = y?=w2829:bool)
                n1731 = Or(x=w2823, y=w2829) -> (x .or. y?=w2822:bool)
                "x = y?" <- w2822
                n1732 = case shown="True" w2822 {
                  selector: w2822 -> [w2839 _]
                  tunnel: w2831 -> [_ _]
                  frame False {
                    n1733 = And(x=w2839, y=TRUE ("Visible")) -> (x .and. y?=w2840:bool)
                    n1734 = property on="message" class="Str"("Visible"=w2840) -> ()  [unwired: 2 in, 2 out]
                  }
                  frame True {
                    n1735 = control-ref of="This VI"() -> (w2851:refnum<vi>)
                    n1736 = property class="VI"(reference=w2851) -> (reference out=w2842:refnum<vi>, error out=w2846:errorcluster, "Panel"=w2850:refnum<vi>)  [unwired: 1 in]
                    n1737 = property on="message" class="Str"("Visible"=FALSE) -> ()  [unwired: 2 in, 2 out]
                    n1738 = property class="Pnl"(reference=w2850, error in=w2846) -> (reference out=w2844:refnum<vi>, error out=w2847:errorcluster, "Panes[]"=w2849:refnum<vi>[])
                    n1739 = for {
                      tunnel: w2849 -> [w2858] mode=indexing
                      tunnel: T21."Always On" ("Horizontal Scrollbar Visibility") -> [w2857]
                      tunnel: w2847 -> [w2854]
                      tunnel: [w2853] -> w2845
                      n1740 = property class="Pane"(reference=w2858, error in=w2854, "HorizScrollbarVisibility"=w2857) -> (reference out=w2855:refnum<vi>, error out=w2856:errorcluster)
                      n1741 = Close Reference(reference=w2855, error in (no error)=w2856) -> (error out=w2853:errorcluster)
                    }
                    n1742 = Close Reference(reference=w2844, error in (no error)=w2845) -> (error out=w2843:errorcluster)
                    n1743 = Close Reference(reference=w2842, error in (no error)=w2843) -> (error out=→"error out 6":errorcluster)
                  }
                }
              }
            }
          }
        }
        n1744 = local read "x = y?"() -> (w2679:bool)
        n1745 = local read "HUMIDITY: 2"() -> (w2681:dbl)
        n1746 = local read "HUMIDITY:"() -> (w2680:dbl)
        n1747 = property on="Port 2 Error" class="Clust (strict)"("Visible"="EDIT") -> ()  [unwired: 2 in, 2 out]
        n1748 = property on="Port 1 Error" class="Clust (strict)"("Visible"="EDIT") -> ()  [unwired: 2 in, 2 out]
        n1749 = case shown="True" "SrvM CP 2" {
          frame False {
          }
          frame True {
            n1750 = local write "SrvM CP 2"(FALSE ("SrvM CP 2")) -> ()
            n1751 = local read "HUMIDITY: 2"() -> (w2720:dbl)
            n1752 = local read "TEMP INTERCEPT: 2"() -> (w2719:dbl)
            n1753 = local read "DISPLACEMENT : 4"() -> (w2723:dbl)
            n1754 = local read "TEMPERATURE : 2"() -> (w2722:dbl)
            n1755 = local read "STROKE GAIN : 2"() -> (w2724:dbl)
            n1756 = local read "FRIC. FORCE : 2"() -> (w2725:dbl)
            n1757 = local read "AIR TEMP INTERCEPT: 2"() -> (w2718:dbl)
            n1758 = local read "AIR TEMPERATURE : 2"() -> (w2721:dbl)
            n1759 = local write "HUMIDITY:"(w2720) -> ()
            n1760 = local write "AIR TEMP INTERCEPT:"(w2719) -> ()
            n1761 = local write "TEMPERATURE :"(w2722) -> ()
            n1762 = local write "FRIC. FORCE :"(w2725) -> ()
            n1763 = local write "STROKE GAIN :"(w2724) -> ()
            n1764 = local write "DISPLACEMENT :"(w2723) -> ()
            n1765 = local write "AIR TEMPERATURE :"(w2721) -> ()
            n1766 = local write "TEMP INTERCEPT:"(w2718) -> ()
          }
        }
        n1767 = Or(x="SAVE", y=w2673) -> (x .or. y?=w2674:bool)
        n1768 = And(x="EDIT", y=w2679) -> (x .and. y?=w2677:bool)
        n1769 = local read "DISPLACEMENT : 4"() -> (w2690:dbl)
        n1770 = local read "TEMPERATURE : 2"() -> (w2688:dbl)
        n1771 = local read "STROKE GAIN : 2"() -> (w2694:dbl)
        n1772 = local read "DISPLACEMENT :"() -> (w2689:dbl)
        n1773 = local read "FRIC. FORCE : 2"() -> (w2697:dbl)
        n1774 = local read "TEMPERATURE :"() -> (w2686:dbl)
        n1775 = local read "STROKE GAIN :"() -> (w2693:dbl)
        n1776 = local read "FRIC. FORCE :"() -> (w2696:dbl)
        n1777 = case shown="True" w2677 {
          tunnel: [u8 2 ("Disabled") u8 0 ("Disabled")] -> w2676
          tunnel: [w3041 TRUE ("Visible")] -> w2675
          frame False {
            w3041 = FALSE ("Visible")
            n1778 = local write "EDIT 2"(w3041) -> ()
          }
          frame True {
          }
        }
        n1779 = case shown="True" w2674 {
          frame False {
          }
          frame True {
            n1780 = stacked-sequence {
              seq-local: [w2889 _ _] -> [_ w3036 _]
              frame #0 {
                (unwired) i16 5 ("precision (6)")
                # "[CH1]    - FF\n[CH2]   - TEMPERATURE\n[CH3]    - Humidity\n[CH4]    - AIR TEMP\n[CH5]\\- Visa Uno\n[CH6] \\- Visa Due\n[CH7]  \\- file path\n[CH8]   - Displacement Gain\n[CHA]   - Stroke Gain\n[CHB]   - Stroke PID Gain\n[CHC]   -Language Selection\n[CHD]   -Power +\n[CHE]   -Power_\n[CHF]   -Heater\n[CHG]   -Humidity Wet\n[CHH]   -Humidity Dry\n[CHI]   -Integral Time"
                n1781 = local read "Language Selection"() -> (w2937:enum16{"English", "Russian"})
                n1782 = local read "CH-HUMIDITY WET"() -> (w2895:u16)
                n1783 = local read "CH-HUMIDITY DRY"() -> (w2892:u16)
                n1784 = local read "STROKE GAIN :"() -> (w2881:dbl)
                n1785 = local read "CH-POWER +"() -> (w2904:u16)
                n1786 = local read "CH-POWER -"() -> (w2901:u16)
                n1787 = local read "CH-HEATER"() -> (w2898:u16)
                n1788 = local read "AIR TEMPERATURE :"() -> (w2884:dbl)
                n1789 = local read "DISPLACEMENT :"() -> (w2882:dbl)
                n1790 = local read "TEMPERATURE :"() -> (w2885:dbl)
                n1791 = local read "FRIC. FORCE :"() -> (w2886:dbl)
                n1792 = local read "HUMIDITY:"() -> (w2883:dbl)
                n1793 = Path To String(path="File Path") -> (string=w2953:string)
                n1794 = Number To Fractional String(number=w2881, width (-)=i16 10 ("precision (6)"), precision (6)=i16 5) -> (F-format string=w2944:string)  [unwired: 1 in]
                n1795 = Number To Fractional String(number=w2937, width (-)=i16 10 ("precision (6)"), precision (6)=i16 5) -> (F-format string=w2933:string)  [unwired: 1 in]
                n1796 = Number To Fractional String(number=w2904, width (-)=i16 10 ("precision (6)"), precision (6)=i16 5) -> (F-format string=w2927:string)  [unwired: 1 in]
                n1797 = Number To Fractional String(number=w2901, width (-)=i16 10 ("precision (6)"), precision (6)=i16 5) -> (F-format string=w2924:string)  [unwired: 1 in]
                n1798 = Number To Fractional String(number=w2898, width (-)=i16 10 ("precision (6)"), precision (6)=i16 5) -> (F-format string=w2919:string)  [unwired: 1 in]
                n1799 = Number To Fractional String(number=w2895, width (-)=i16 10 ("precision (6)"), precision (6)=i16 5) -> (F-format string=w2916:string)  [unwired: 1 in]
                n1800 = Number To Fractional String(number=w2892, width (-)=i16 10 ("precision (6)"), precision (6)=i16 5) -> (F-format string=w2911:string)  [unwired: 1 in]
                n1801 = local read "Com Port 1"() -> (w2888:refnum<visa-resource-name>)
                n1802 = local read "Com Port 2"() -> (w2887:refnum<visa-resource-name>)
                n1803 = Concatenate Strings(w2953, "\\" ("string")) -> (w2952:string)
                n1804 = Number To Fractional String(number=w2886, width (-)=i16 10 ("precision (6)"), precision (6)=i16 5) -> (F-format string=w2985:string)  [unwired: 1 in]
                n1805 = Number To Fractional String(number=w2885, width (-)=i16 10 ("precision (6)"), precision (6)=i16 5) -> (F-format string=w2984:string)  [unwired: 1 in]
                n1806 = Number To Fractional String(number=w2883, width (-)=i16 10 ("precision (6)"), precision (6)=i16 5) -> (F-format string=w2978:string)  [unwired: 1 in]
                n1807 = Number To Fractional String(number=w2884, width (-)=i16 10 ("precision (6)"), precision (6)=i16 5) -> (F-format string=w2972:string)  [unwired: 1 in]
                n1808 = Number To Fractional String(number=w2882, width (-)=i16 10 ("precision (6)"), precision (6)=i16 5) -> (F-format string=w2945:string)  [unwired: 1 in]
                n1809 = Concatenate Strings("[CHA]" ("string"), w2944, "- Stroke Gain" ("string"), "\r") -> (w2938:string)
                n1810 = Concatenate Strings("[CHC]" ("string"), w2933, "-Language Selection" ("string"), "\r") -> (w2930:string)
                n1811 = Concatenate Strings("[CHD]" ("string"), w2927, "-Power +" ("string"), "\r") -> (w2909:string)
                n1812 = Concatenate Strings("[CHG]" ("string"), w2916, "-Humidity Wet" ("string"), "\r") -> (w2906:string)
                n1813 = Concatenate Strings("[CHH]" ("string"), w2911, "-Humidity Dry" ("string"), "\r") -> (w2905:string)
                n1814 = Concatenate Strings("[CH1]" ("string"), w2985, " - FF" ("string"), "\r") -> (w2983:string)
                n1815 = Concatenate Strings("[CH2]" ("string"), w2984, " - TEMPERATURE" ("string"), "\r") -> (w2982:string)
                n1816 = Concatenate Strings("[CH3]" ("string"), w2978, " - Humidity" ("string"), "\r") -> (w2975:string)
                n1817 = Concatenate Strings("[CH4]" ("string"), w2972, " - AIR TEMP" ("string"), "\r") -> (w2968:string)
                n1818 = Concatenate Strings("[CH5]" ("string"), w2888, "- Visa Uno" ("string"), "\r") -> (w2961:string)
                n1819 = Concatenate Strings("[CH6]" ("string"), w2887, "- Visa Due" ("string"), "\r") -> (w2956:string)
                n1820 = Concatenate Strings("[CH7]" ("string"), w2952, "- file path" ("string"), "\r") -> (w2955:string)
                n1821 = Concatenate Strings("[CH8]" ("string"), w2945, "- Displacement Gain" ("string"), "\r") -> (w2948:string)
                n1822 = Concatenate Strings("[CHE]" ("string"), w2924, "-Power_" ("string"), "\r") -> (w2908:string)
                n1823 = Concatenate Strings("[CHF]" ("string"), w2919, "-Heater" ("string"), "\r") -> (w2907:string)
                n1824 = Concatenate Strings(w2983, w2982, w2975, w2968, w2961, w2956, w2955, w2948, w2938, w2930, w2909, w2908, w2907, w2906, w2905) -> (w2889:string)
                "gain" <- w2889
              }
              frame #1 {
                n1825 = local read "Camera Port :"() -> (w2997:string)
                n1826 = local read "C3 :"() -> (w3005:refnum<visa-resource-name>)
                n1827 = local read "TEMP INTERCEPT:"() -> (w3006:dbl)
                n1828 = local read "AIR TEMP INTERCEPT:"() -> (w3007:dbl)
                n1829 = local read "Com Port 3"() -> (w3008:refnum<visa-resource-name>)
                n1830 = Concatenate Strings("[CH8]" ("string"), w2997, "- Visa Camera" ("string"), "\r") -> (w2996:string)
                n1831 = Concatenate Strings("[CH7]" ("string"), w3005, "- Visa Humidity" ("string"), "\r") -> (w3001:string)
                n1832 = Number To Fractional String(number=w3006, width (-)=i16 10 ("precision (6)"), precision (6)=i16 5) -> (F-format string=w3024:string)  [unwired: 1 in]
                n1833 = Concatenate Strings("[CHL]" ("string"), w3008, "- Visa humid" ("string"), "\r") -> (w3011:string)
                n1834 = Number To Fractional String(number=w3007, width (-)=i16 10 ("precision (6)"), precision (6)=i16 5) -> (F-format string=w3031:string)  [unwired: 1 in]
                n1835 = Concatenate Strings("[CHK]" ("string"), w3024, "-TEMP INTERCEPT" ("string"), "\r") -> (w3020:string)
                n1836 = Concatenate Strings("[SNO]" ("string"), "S.NO", "-" ("string"), "\r") -> (w3016:string)
                n1837 = Concatenate Strings("[CHJ]" ("string"), w3031, "-AIR TEMP INTERCEPT" ("string"), "\r") -> (w3021:string)
                n1838 = String To Path(string="C:\\LAB-IQ\\calibrate WO 2465.dcf") -> (path=w3009:path)
                n1839 = Concatenate Strings(w3036, w3021, w3020, w3016, w3011, w3001, w2996) -> (w3035:string)
                n1840 = call <vilib>:"Write Characters To File.vi"("append to file? (new file:F)"=FALSE, "character string"=w3035, "file path (dialog if empty)"=w3009) -> ()  [unwired: 2 in, 1 out]
              }
              frame #2 {
                n1841 = local write "Lan flag"(0.0 ("Lan flag")) -> ()
                n1842 = local write "conststatus"(0.0 ("rpm value : 2")) -> ()
                n1843 = local write "SAVE"(FALSE ("OK Button 14")) -> ()
                n1844 = local write "SAVE 2"(FALSE ("SAVE 2")) -> ()
              }
            }
          }
        }
        n1845 = Subtract(x=w2681, y=w2680) -> (x-y=w2682:dbl)
        n1846 = local read "AIR TEMPERATURE : 2"() -> (w2685:dbl)
        n1847 = local read "AIR TEMPERATURE :"() -> (w2684:dbl)
        n1848 = Divide(x=w2682, y=w2680) -> (x/y=w2704:dbl)
        n1849 = Subtract(x=w2697, y=w2696) -> (x-y=w2695:dbl)
        n1850 = Subtract(x=w2688, y=w2686) -> (x-y=w2687:dbl)
        n1851 = Subtract(x=w2694, y=w2693) -> (x-y=w2692:dbl)
        n1852 = Subtract(x=w2690, y=w2689) -> (x-y=w2691:dbl)
        n1853 = Subtract(x=w2685, y=w2684) -> (x-y=w2683:dbl)
        n1854 = Divide(x=w2695, y=w2696) -> (x/y=w2715:dbl)
        n1855 = Divide(x=w2687, y=w2686) -> (x/y=w2708:dbl)
        n1856 = Divide(x=w2692, y=w2693) -> (x/y=w2712:dbl)
        n1857 = Divide(x=w2691, y=w2689) -> (x/y=w2711:dbl)
        n1858 = Multiply(x=w2704, y=100.0) -> (x*y=→"HUMIDITY  Calibration Error":dbl)
        n1859 = Divide(x=w2683, y=w2684) -> (x/y=w2707:dbl)
        n1860 = Multiply(x=w2715, y=100.0) -> (x*y=→"FRIC. FORCE Calibration Error":dbl)
        n1861 = Multiply(x=w2708, y=100.0) -> (x*y=→"TEMPERATURE  Calibration Error":dbl)
        n1862 = Multiply(x=w2712, y=100.0) -> (x*y=→"STROKE Calibration Error":dbl)
        n1863 = Multiply(x=w2711, y=100.0) -> (x*y=→"DISPLACEMENT  Calibration Error":dbl)
        n1864 = property on="EDIT 2" class="Bool (strict)"("Visible"=w2675) -> ()  [unwired: 2 in, 2 out]
        n1865 = property on="SAVE" class="Bool (strict)"("Visible"=w2675) -> ()  [unwired: 2 in, 2 out]
        n1866 = property on="SrvM CP" class="Bool (strict)"("Disabled"=w2676) -> ()  [unwired: 2 in, 2 out]
        n1867 = property on="visa due" class="CmbBox"("Disabled"=w2676) -> ()  [unwired: 2 in, 2 out]
        n1868 = property on="File Path" class="Path"("Disabled"=w2676) -> ()  [unwired: 2 in, 2 out]
        n1869 = Multiply(x=w2707, y=100.0) -> (x*y=→"AIR TEMPERATURE  Calibration Error":dbl)
        n1870 = property on="Language Selection" class="Enum (strict)"("Visible"=w2675) -> ()  [unwired: 2 in, 2 out]
        n1871 = property on="Tab Control 7" class="TabCtl (strict)"("Disabled"=w2676) -> ()  [unwired: 2 in, 2 out]
        n1872 = property on="AIR TEMP INTERCEPT:" class="DigNum (strict)"("Disabled"=w2676) -> ()  [unwired: 2 in, 2 out]
        n1873 = property on="CH-POWER -" class="DigNum (strict)"("Disabled"=w2676) -> ()  [unwired: 2 in, 2 out]
        n1874 = property on="CH-POWER +" class="DigNum (strict)"("Disabled"=w2676) -> ()  [unwired: 2 in, 2 out]
        n1875 = property on="AIR TEMPERATURE :" class="DigNum (strict)"("Disabled"=w2676) -> ()  [unwired: 2 in, 2 out]
        n1876 = property on="STROKE GAIN :" class="DigNum (strict)"("Disabled"=w2676) -> ()  [unwired: 2 in, 2 out]
        n1877 = property on="SPEED OUT:" class="DigNum (strict)"("Disabled"=w2676) -> ()  [unwired: 2 in, 2 out]
        n1878 = property on="CH-HUMIDITY DRY" class="DigNum (strict)"("Disabled"=w2676) -> ()  [unwired: 2 in, 2 out]
        n1879 = property on="HUMIDITY:" class="DigNum (strict)"("Disabled"=w2676) -> ()  [unwired: 2 in, 2 out]
        n1880 = property on="CH-HUMIDITY WET" class="DigNum (strict)"("Disabled"=w2676) -> ()  [unwired: 2 in, 2 out]
        n1881 = property on="TEMPERATURE :" class="DigNum (strict)"("Disabled"=w2676) -> ()  [unwired: 2 in, 2 out]
        n1882 = property on="DISPLACEMENT :" class="DigNum (strict)"("Disabled"=w2676) -> ()  [unwired: 2 in, 2 out]
        n1883 = property on="CH-HEATER" class="DigNum (strict)"("Disabled"=w2676) -> ()  [unwired: 2 in, 2 out]
        n1884 = property on="TEMP INTERCEPT:" class="DigNum (strict)"("Disabled"=w2676) -> ()  [unwired: 2 in, 2 out]
        n1885 = property on="FRIC. FORCE :" class="DigNum (strict)"("Disabled"=w2676) -> ()  [unwired: 2 in, 2 out]
      }
    }
    n1886 = local read "RUN"() -> (w2070:bool)
    n1887 = local read "RUN"() -> (w2068:bool)
    n1888 = disable-structure shown="Disabled" {
      disable-tunnel: [w2085 _] -> w2051
      disable-tunnel: [w2084 _] -> w2049
      frame Disabled {
        n1889 = local read "Temperature before test"() -> (w2078:dbl)
        n1890 = local read "Temperature after test"() -> (w2091:dbl)
        n1891 = case shown="True" "Save Results" {
          frame False {
          }
          frame True {
            w2107 = "\r"
            n1892 = local write "Save Results"(FALSE ("OK Button 5")) -> ()
            n1893 = local read "Temperature before test"() -> (w2145:dbl)
            n1894 = local read "Temperature after test"() -> (w2147:dbl)
            n1895 = local read "Humidity before test"() -> (w2144:dbl)
            n1896 = local read "Humidity after test"() -> (w2146:dbl)
            n1897 = local read "WS1.4"() -> (w2151:dbl)
            n1898 = local read "AVP"() -> (w2149:dbl)
            n1899 = Number To Fractional String(number=w2151, width (-)=i16 6, precision (6)=i16 1) -> (F-format string=w2111:string)  [unwired: 1 in]
            n1900 = local read "MWSD"() -> (w2148:dbl)
            n1901 = local read "String"() -> (w2140:string)
            n1902 = local read "FILE"() -> (w2143:string)
            n1903 = local read "HCF"() -> (w2150:dbl)
            n1904 = Number To Fractional String(number=w2144, width (-)=i16 6, precision (6)=i16 1) -> (F-format string=w2136:string)  [unwired: 1 in]
            n1905 = Number To Fractional String(number=w2145, width (-)=i16 6, precision (6)=i16 1) -> (F-format string=w2133:string)  [unwired: 1 in]
            n1906 = Number To Fractional String(number=w2146, width (-)=i16 6, precision (6)=i16 1) -> (F-format string=w2129:string)  [unwired: 1 in]
            n1907 = Number To Fractional String(number=w2147, width (-)=i16 6, precision (6)=i16 1) -> (F-format string=w2125:string)  [unwired: 1 in]
            n1908 = Number To Fractional String(number=w2149, width (-)=i16 6, precision (6)=i16 3) -> (F-format string=w2118:string)  [unwired: 1 in]
            n1909 = Concatenate Strings(w2140, w2143) -> (w2162:string)
            n1910 = Number To Fractional String(number=w2148, width (-)=i16 6, precision (6)=i16 1) -> (F-format string=w2122:string)  [unwired: 1 in]
            n1911 = Number To Fractional String(number=w2150, width (-)=i16 6, precision (6)=i16 2) -> (F-format string=w2116:string)  [unwired: 1 in]
            n1912 = Concatenate Strings("(" ("string"), w2111, ")Microns" ("string")) -> (w2110:string)
            n1913 = local read "REMARKS"() -> (w2142:string)
            "REMARKS 2" <- w2142
            n1914 = Concatenate Strings("(" ("string"), w2136, " ) % RH," ("string")) -> (w2137:string)
            n1915 = Concatenate Strings(w2116, ")" ("string")) -> (w2114:string)
            n1916 = Concatenate Strings("(" ("string"), w2133, ")  Deg C ," ("string")) -> (w2132:string)
            n1917 = Concatenate Strings("(" ("string"), w2129, " ) % RH," ("string")) -> (w2128:string)
            n1918 = Concatenate Strings("(" ("string"), w2125, ")  Deg C ," ("string")) -> (w2124:string)
            n1919 = Concatenate Strings("(" ("string"), w2122, ")  Microns," ("string")) -> (w2121:string)
            n1920 = Concatenate Strings("(" ("string"), w2118, ")  kPa," ("string")) -> (w2108:string)
            n1921 = Concatenate Strings(w2162, ".dwm" ("Substring")) -> (w2160:string)
            n1922 = String To Path(string=w2160) -> (path=w2159:path)
            n1923 = Concatenate Strings(w2142, w2107, " Humidity before test= " ("Substring"), w2137, w2107, " Temperature before test = " ("Substring"), w2132, w2107, " Humidity after test= " ("Substring"), w2128, w2107, "Temperature after test = " ("Substring"), w2124, w2107, "MSD = " ("Substring"), w2121, w2107, "  AVP = " ("Substring"), w2108, w2107, "  HCF                     =( " ("Substring"), w2114, w2107, " WS1.4                  = " ("Substring"), w2110, w2107) -> (w2106:string)
            "data" <- w2106
            n1924 = call <vilib>:"Write Characters To File.vi"("append to file? (new file:F)"=FALSE, "character string"=w2106, "file path (dialog if empty)"=w2159) -> ()  [unwired: 2 in, 1 out]
            n1925 = Match Pattern(string=w2106, regular expression="!") -> (after substring=→"export":string)  [unwired: 1 in, 3 out]
          }
        }
        n1926 = Add(x=231.864, y=w2078) -> (x+y=w2075:dbl)
        n1927 = Add(x=231.864, y=w2091) -> (x+y=w2088:dbl)
        n1928 = Divide(x=1705.984, y=w2075) -> (x/y=w2076:dbl)
